vi "LineFollower.vi"   [LabVIEW 2016, in "Moving Motor.lvrbt"]
uses:
  Moving Motor.lvrbt
  <vilib>/NXT/Hardware/Plugins/Tetrix DC Motor/TetrixDCMotorAddress.ctl
  <vilib>/NXT/Block Support/NXT_InputPort.ctl
  <vilib>/NXT/NXTIO Xnodes/NXTIONodeSubVIs/TETRIX IO Move DC Motors.vi
  <vilib>/NXT/Dual Mode Library/Sensors/EV3_Color_Reflect.vi
  <vilib>/NXT/Subs/LVHSConnector.ctl
  <vilib>/NXT/NXTIO Xnodes/AddressXNode/NXTIOAddress.xnode
  <vilib>/NXT/NXTIO Xnodes/NXTIOXNode/NXTIO.xnode
  <vilib>/NXT/LegoClasses/BrickReference/BrickReference.lvclass
types:
  T1 = typedef "TetrixDCMotorAddress.ctl" = i32
  T2 = typedef "LVHSConnector.ctl" = refnum<class "BrickReference.lvclass">
  T3 = cluster{"TetrixDCMotor":T1, "TetrixDCMotor 2":T1}
  T4 = typedef "NXT_InputPort.ctl" = u32
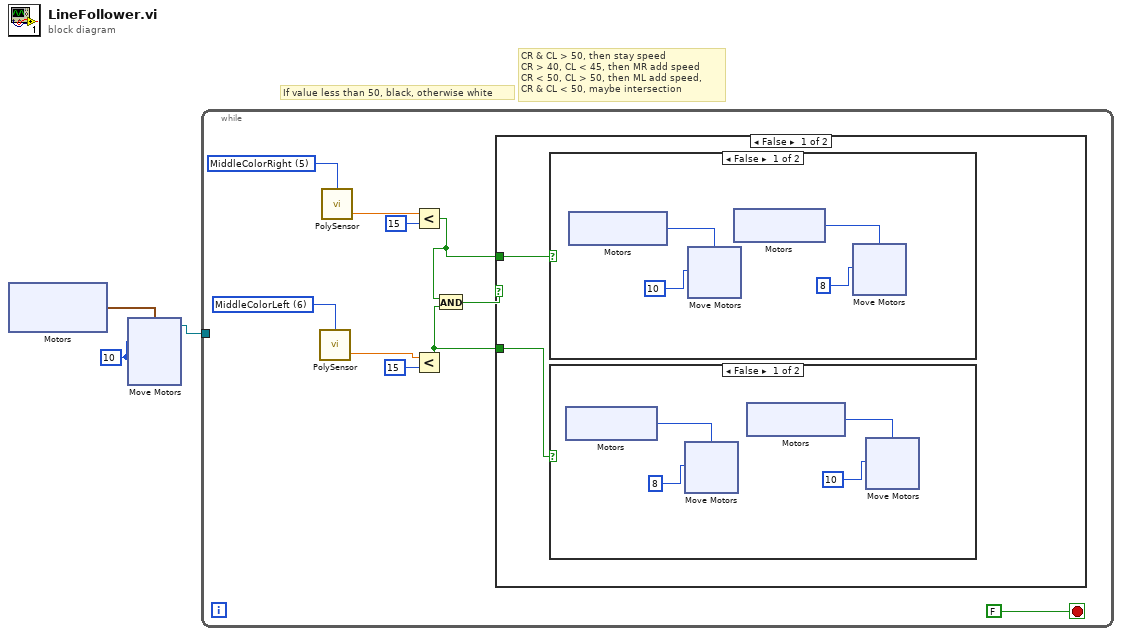
[diagram p0: block diagram]
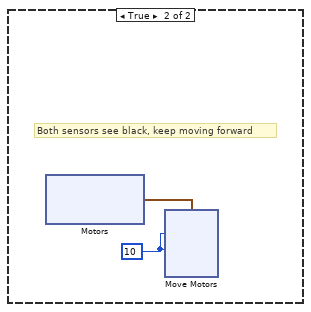
[diagram p4: hidden frame]
diagram:
  w3 = i8 10 ("Power/Speed 2")
  # "CR & CL > 50, then stay speed\nCR > 40, CL < 45, then MR add speed\nCR < 50, CL > 50, then ML add speed,\nCR & CL < 50, maybe intersection"
  # "If value less than 50, black, otherwise white"
  n1 = xnode "Motors"() -> ("Motor"=w2:cluster{"TetrixDCMotor":T1, "TetrixDCMotor":T1})
  n2 = xnode "Move Motors"("Power/Speed 2"=w3, "Power/Speed 1"=w3, "Motors"=w2) -> ("NXT/EV3"=w1:T2)  [unwired: 1 in]
  n3 = while {
    tunnel: w1 -> [_]
    stop <- FALSE stop-if-true
    w11 = T4 6 items=["Port 1"=0, "Port 2"=1, "Port 3"=2, "Port 4"=3, "MiddleColorLeft"=6] ("ColorLeft")
    w12 = T4 5 items=["Port 1"=0, "Port 2"=1, "Port 3"=2, "Port 4"=3, "MiddleColorRight"=5] ("ColorRight")
    n4 = call-poly <vilib>:"PolySensor.vi"("Port (Port 1)"=w11) -> ("Scaled Value"=w7:sgl)  [unwired: 2 in, 1 out]
    n5 = call-poly <vilib>:"PolySensor.vi"("Port (Port 1)"=w12) -> ("Scaled Value"=w10:sgl)  [unwired: 2 in, 1 out]
    n6 = Less?(x=w10, y=i16 15) -> (x < y?=w5:bool)
    n7 = Less?(x=w7, y=i16 15) -> (x < y?=w4:bool)
    n8 = And(x=w5, y=w4) -> (x .and. y?=w6:bool)
    n9 = case "Case 1 and 4" shown="False" w6 {
      tunnel: w5 -> [w15 _]
      tunnel: w4 -> [w14 _]
      frame False {
        n10 = case shown="False" w15 {
          frame False {
            n11 = xnode "Motors"() -> ("Motor"=w38:T1)
            n12 = xnode "Move Motors"("Power/Speed 1"=i8 10 ("Power/Speed 2"), "Motors"=w38) -> ()  [unwired: 1 in, 1 out]
            n13 = xnode "Motors"() -> ("Motor"=w36:T1)
            n14 = xnode "Move Motors"("Power/Speed 1"=i8 8 ("Power/Speed 2"), "Motors"=w36) -> ()  [unwired: 1 in, 1 out]
          }
          frame True {
          }
        }
        n15 = case shown="False" w14 {
          frame False {
            n16 = xnode "Motors"() -> ("Motor"=w19:T1)
            n17 = xnode "Move Motors"("Power/Speed 1"=i8 8 ("Power/Speed 2"), "Motors"=w19) -> ()  [unwired: 1 in, 1 out]
            n18 = xnode "Motors"() -> ("Motor"=w17:T1)
            n19 = xnode "Move Motors"("Power/Speed 1"=i8 10 ("Power/Speed 2"), "Motors"=w17) -> ()  [unwired: 1 in, 1 out]
          }
          frame True {
          }
        }
      }
      frame True {
        w56 = i8 10 ("Power/Speed 2")
        # "Both sensors see black, keep moving forward"
        n20 = xnode "Motors"() -> ("Motor"=w57:cluster{"TetrixDCMotor":T1, "TetrixDCMotor":T1})
        n21 = xnode "Move Motors"("Power/Speed 2"=w56, "Power/Speed 1"=w56, "Motors"=w57) -> ()  [unwired: 1 in, 1 out]
      }
    }
  }
